vi "oa_Calculate Interpolation Filter Delay Length.vi"(1 "filter info input":cluster{"filter length":i32, "factor":i32}[](array[cluster])) -> (0 "delay length":i32)   [LabVIEW 2017, in "SoundVib_Resampling.lvlib"]
uses:
  <vilib>/addons/Sound and Vibration/Order Analysis/Resample Order Tracking/SoundVib_Resampling.lvlib
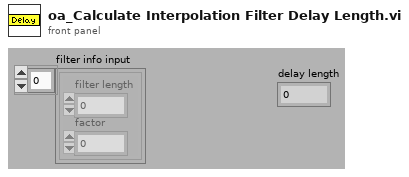
[diagram p1: front panel]
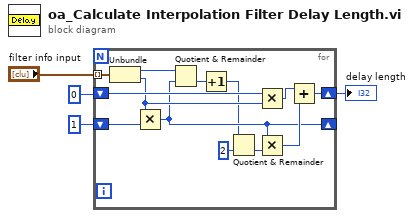
[diagram p0: block diagram]
diagram:
  n1 = for {
    tunnel: "filter info input" -> [w16] mode=indexing
    shift-right: [w11] -> w2
    shift-left: 0 -> [w14]
    shift-right: [w8] -> _
    shift-left: 1 -> [w10]
    n2 = Unbundle(w16) -> ("filter length"=w15:i32, "factor"=w9:i32)
    n3 = Multiply(x=w9, y=w10) -> (x*y=w8:i32)
    n4 = Quotient & Remainder(x=w15, y=w8) -> (floor(x/y)=w7:i32)  [unwired: 1 out]
    n5 = Increment(x=w7) -> (x+1=w5:i32)
    n6 = Quotient & Remainder(x=w5, y=2) -> (floor(x/y)=w6:i32)  [unwired: 1 out]
    n7 = Multiply(x=w14, y=w9) -> (x*y=w13:i32)
    n8 = Multiply(x=w8, y=w6) -> (x*y=w12:i32)
    n9 = Add(x=w13, y=w12) -> (x+y=w11:i32)
  }
  "delay length" <- w2
